vi "WilliamPI_CameraRead MJPG for Dashboard.vi"(6 "Camera Settings":T2={"fps"=30, "compression"=30, "Image Size"=enum."320x240"}, 8 "Rec Mode":u16(ring) items=["O", "*", "Open Playback Panel"], 9 "Camera IP":string, 10 "Camera Mode":u16(ring) items=["Camera Off", "USB Camera SW", "USB Camera HW", "IP Camera"], 11 "Refnum in":T1) -> (2 "Active":bool, 3 "Refnum out":T1, 4 "FPS":dbl, 5 "Bandwidth (Mbps)":dbl)   [LabVIEW 2015]
uses:
  <vilib>/Rock Robotics/WPI/Camera/WPI_CameraSettings Read MJPG.ctl
  <vilib>/Rock Robotics/WPI/Camera/WPI_CameraImageSize.ctl
  <vilib>/vision/Image Controls.llb/IMAQ Image.ctl
  <vilib>/Rock Robotics/WPI/Dashboard/WPI_DashboardLogging Global.vi
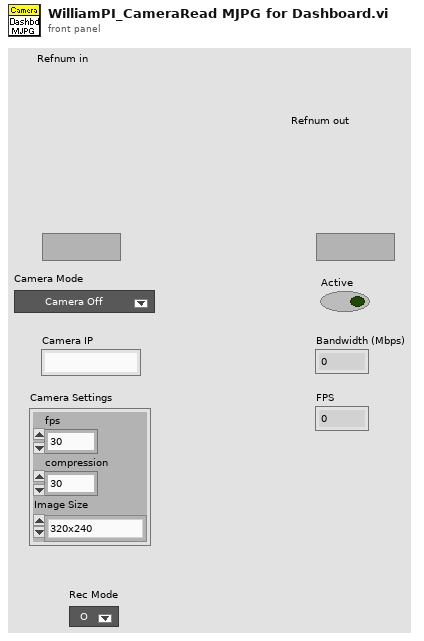
[diagram p1: front panel]
types:
  T1 = typedef "IMAQ Image.ctl" = refnum<image>
  T2 = typedef "WPI_CameraSettings Read MJPG.ctl" = cluster{"fps":i32, "compression":i32, "Image Size":T3}
  T3 = typedef "WPI_CameraImageSize.ctl" = enum16{"640x480", "320x240", "160x120", "Custom"}
  T4 = typedef "IMAQ AVI2 Refnum.ctl" = refnum<k20>
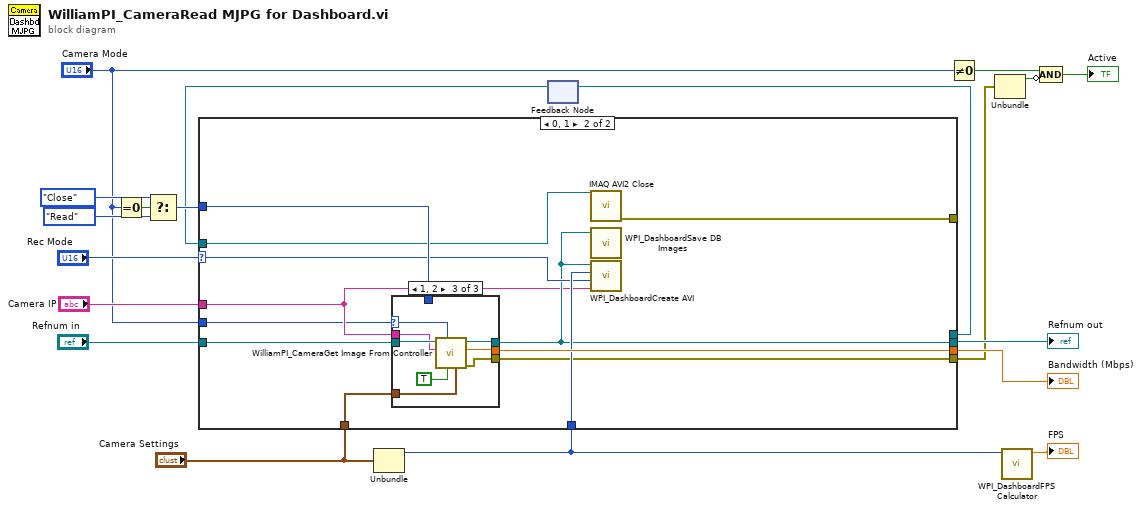
[diagram p0: block diagram]
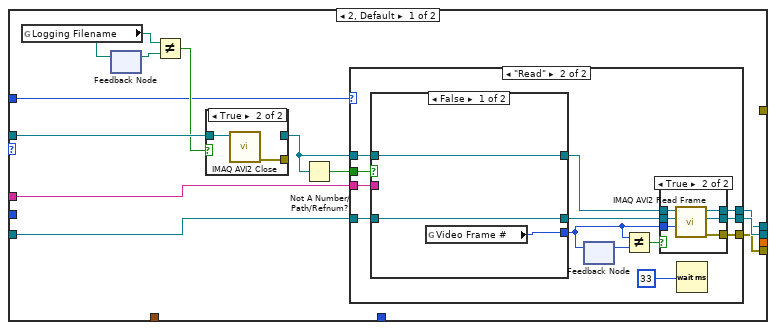
[diagram p2: hidden frame]
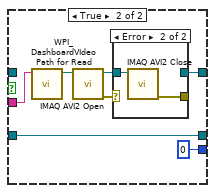
[diagram p5: hidden frame]
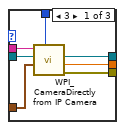
[diagram p8: hidden frame]
diagram:
  n1 = Equal To 0?(x="Camera Mode") -> (x = 0?=w3:bool)
  n2 = Select(t=enum16{"Read", "Reopen", "Close"}."Close" ("Operation"), s=w3, f=enum16{"Read", "Reopen", "Close"}."Read" ("Operation")) -> (s? t:f=w15:enum16{"Read", "Reopen", "Close"})
  n3 = Unbundle("Camera Settings") -> ("fps"=w7:i32)  [unwired: 2 out]
  n4 = feedback #1() -> (w6:T4)  [unwired: 1 in]
  n5 = case shown="0, 1" "Rec Mode" {
    selector: "Rec Mode" -> [_ w77]
    tunnel: "Camera Settings" -> [_ w82]
    tunnel: w15 -> [w20 w81]
    tunnel: [_ w80] -> w12
    tunnel: [w31 w73] -> w8
    tunnel: "Refnum in" -> [w29 w79]
    tunnel: "Camera IP" -> [w26 w72]
    tunnel: w7 -> [_ w78]
    tunnel: w6 -> [w24 w75]
    tunnel: [w28 _] -> w5
    tunnel: [w27 w76] -> w4
    tunnel: [_ w74] -> _
    tunnel: "Camera Mode" -> [_ w71]
    frame 2, Default {
      n6 = global read "WPI_DashboardLogging Global.vi" "Logging Filename"() -> (w23:path)
      n7 = feedback #2() -> (w22:path)  [unwired: 1 in]
      n8 = feedback-in #2(w23) -> ()
      n9 = Not Equal?(x=w23, y=w22) -> (x != y?=w21:bool)
      n10 = case shown="True" w21 {
        tunnel: [w68 _] -> w25
        tunnel: w24 -> [w68 w70]
        tunnel: [_ w69] -> _
        frame False {
        }
        frame True {
          n11 = call "IMAQ AVI2 Close"("AVI Refnum"=w70) -> ("error out"=w69:errorcluster)  [unwired: 10 in]
        }
      }
      n12 = Not A Number/Path/Refnum?(number/path/refnum=w25) -> (NaN/Path/Refnum?=w30:bool)
      n13 = case shown="\"Read\"" w20 {
        tunnel: [w32 w46] -> w31
        tunnel: w30 -> [_ w45]
        tunnel: w29 -> [w32 w42]
        tunnel: [w33 w41] -> w28
        tunnel: [_ w40] -> w27
        tunnel: w26 -> [_ w39]
        tunnel: w25 -> [w33 w38]
        frame "Close", Default {
        }
        frame "Read" {
          n14 = case shown="False" w45 {
            tunnel: [w57 w62] -> w44
            tunnel: w38 -> [w57 _]
            tunnel: [w56 w64] -> w43
            tunnel: w42 -> [w56 w64]
            tunnel: [w55 0 ("Video Frame #")] -> w35
            tunnel: w39 -> [_ w59]
            frame False {
              n15 = global read "WPI_DashboardLogging Global.vi" "Video Frame #"() -> (w55:i32)
            }
            frame True {
              n16 = call <vilib>:"WPI_DashboardVIdeo Path for Read.vi"("Camera IP"=w59) -> ("Video Path"=w58:path)  [unwired: 10 in]
              n17 = call "IMAQ AVI2 Open"("AVI File Path"=w58) -> ("error out"=w63:errorcluster, "AVI Refnum"=w61:T4)  [unwired: 9 in]
              n18 = case shown="Error" w63 {
                tunnel: [w65 _] -> w62
                tunnel: w61 -> [w65 w67]
                tunnel: [_ w66] -> _
                frame No Error {
                }
                frame Error {
                  n19 = call "IMAQ AVI2 Close"("AVI Refnum"=w67) -> ("error out"=w66:errorcluster)  [unwired: 10 in]
                }
              }
            }
          }
          n20 = feedback #3() -> (w36:i32)  [unwired: 1 in]
          n21 = feedback-in #3(w35) -> ()
          n22 = Not Equal?(x=w35, y=w36) -> (x != y?=w37:bool)
          n23 = case shown="True" w37 {
            tunnel: [w47 w54] -> w46
            tunnel: w44 -> [w48 w53]
            tunnel: w43 -> [w47 w52]
            tunnel: [w48 w51] -> w41
            tunnel: [_ w50] -> w40
            tunnel: w35 -> [_ w49]
            frame False {
            }
            frame True {
              n24 = call "IMAQ AVI2 Read Frame"("Frame Number"=w49, "Image"=w52, "AVI Refnum"=w53) -> ("error out"=w50:errorcluster, "Image Out"=w54:T1, "AVI Refnum (duplicate)"=w51:T4)  [unwired: 6 in]
            }
          }
          n25 = Wait (ms)(milliseconds to wait=33) -> ()  [unwired: 1 out]
        }
      }
    }
    frame 0, 1 {
      n26 = case shown="1, 2" w71 {
        selector: w71 -> [_ _ w98]
        tunnel: w82 -> [w89 _ w92]
        tunnel: w81 -> [w83 _ _]
        tunnel: [w87 _ w95] -> w80
        tunnel: w79 -> [w85 w90 w97]
        tunnel: w72 -> [w84 _ w91]
        tunnel: [w88 _ w94] -> w76
        tunnel: [w86 w90 w96] -> w73
        frame 3 {
          n27 = call <vilib>:"WPI_CameraDirectly from IP Camera.vi"("Operation"=w83, "Camera Settings"=w89, "Image"=w85, "address"=w84) -> ("error out"=w88:errorcluster, "Bandwidth (Mbps)"=w87:dbl, "Image Out"=w86:T1)  [unwired: 5 in]
        }
        frame Default {
        }
        frame 1, 2 {
          n28 = call "WilliamPI_CameraGet Image From Controller.vi"("Camera Settings"=w92, "USB"=TRUE, "Camera Mode"=w98, "Controller Address"=w91, "Image"=w97) -> ("error out"=w94:errorcluster, "Bandwidth (Mbps)"=w95:dbl, "Image Out"=w96:T1)  [unwired: 4 in]
        }
      }
      n29 = call "IMAQ AVI2 Close"("AVI Refnum"=w75) -> ("error out"=w74:errorcluster)  [unwired: 10 in]
      n30 = call <vilib>:"WPI_DashboardSave DB Images.vi"("Image"=w73) -> ()  [unwired: 3 in]
      n31 = call <vilib>:"WPI_DashboardCreate AVI.vi"("Camera IP"=w72, "Recording"=w77, "frames per seconds"=w78, "Image"=w73) -> ()  [unwired: 8 in]
    }
  }
  "Bandwidth (Mbps)" <- w12
  "Refnum out" <- w8
  n32 = feedback-in #1(w5) -> ()
  n33 = Not Equal To 0?(x="Camera Mode") -> (x != 0?=w2:bool)
  n34 = Unbundle(w4) -> ("status"=w16:bool)  [unwired: 2 out]
  n35 = call <vilib>:"WPI_DashboardFPS Calculator.vi"("Average Count"=w7) -> ("fps"=→"FPS":dbl)  [unwired: 10 in]
  n36 = Compound Arithmetic op=AND(w2, invert w16) -> (→"Active":bool)
